vi "Define_Indicies_for_Subtracks_Cost_F()-1.vi"(2 "[IN] Number of Rows":i32, 3 "[IN] Current index":i32) -> (0 "[OUT] Column \n# for Subtrack":i32, 1 "[OUT] Row # \nfor Subtrack":i32)   [LabVIEW 2013]
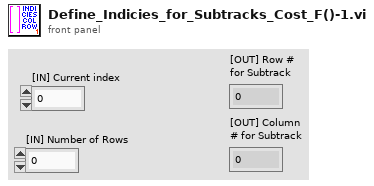
[diagram p1: front panel]
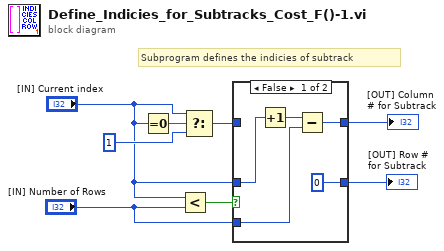
[diagram p0: block diagram]
diagram:
  # "Subprogram defines the indicies of subtrack"
  n1 = Equal To 0?(x="[IN] Current index") -> (x = 0?=w8:bool)
  n2 = Less?(x="[IN] Current index", y="[IN] Number of Rows") -> (x < y?=w6:bool)
  n3 = Select(t="[IN] Current index", s=w8, f=1) -> (s? t:f=w5:i32)
  n4 = case shown="False" w6 {
    tunnel: w5 -> [_ w15]
    tunnel: [w9 w15] -> w4
    tunnel: "[IN] Current index" -> [w11 w14]
    tunnel: [0 ("disabled index (row)") w14] -> w2
    tunnel: "[IN] Number of Rows" -> [w10 _]
    frame False {
      n5 = Increment(x=w11) -> (x+1=w12:i32)
      n6 = Subtract(x=w12, y=w10) -> (x-y=w9:i32)
    }
    frame True {
    }
  }
  "[OUT] Column \n# for Subtrack" <- w4
  "[OUT] Row # \nfor Subtrack" <- w2
